vi "Export_TimeDomain_Data.vi"(0 "nCmdShow":i16(ring) items=["SW_HIDE   ", "SW_SHOWNORMAL", "SW_SHOWMINIMIZED", "SW_SHOWMAXIMIZED", "SW_SHOWNOACTIVATE", "SW_SHOW", "SW_MINIMIZE", "SW_SHOWMINNOACTIVE", "SW_SHOWNA", "SW_RESTORE"], 1 "szFileName":string="D:\\TX1.s4p", 2 "delimiterType":i16(ring) items=["Tab", "Comma"], 3 "dataFormat":i16(ring)=2 items=["StepReal", "ImpulseReal", "StepVolts", "ImpulseVolts", "StepLog", "ImpulseLog", "StepImpedance"], 4 "dataToExport":i16(ring)=3 items=["SE", "Balanced", "All ", "Customized"], 5 "stopTimeNs":dbl=3.0, 6 "ParamList":string="TDD11,TDD22", 7 "Data Points":i32=4000, 8 "Port Type":u16(ring)=1, 9 "startTimeNs":dbl, 10 "Filter?":bool, 11 "FileName":string="D:\\data.txt", 12 "Filter Risetime(ps)":dbl=50.0 min=1.0 max=1000.0 step=1.0, 13 "Compensation(ohm)":dbl=0.001 min=-20.0 max=20.0 step=0.1, 15 "Index":i32) -> (20 "Data Out":dbl[][](array[numeric]), 23 "Time Array":dbl[](array[numeric]))   [LabVIEW 2011]
uses:
  Data/Interop.PLTS.dll
  <vilib>/Utility/file.llb/Read From Spreadsheet File (DBL).vi
panel:
  out "Find?":bool=TRUE
  out "Impedance Chart":cluster{dbl[], dbl[]}[](graph)
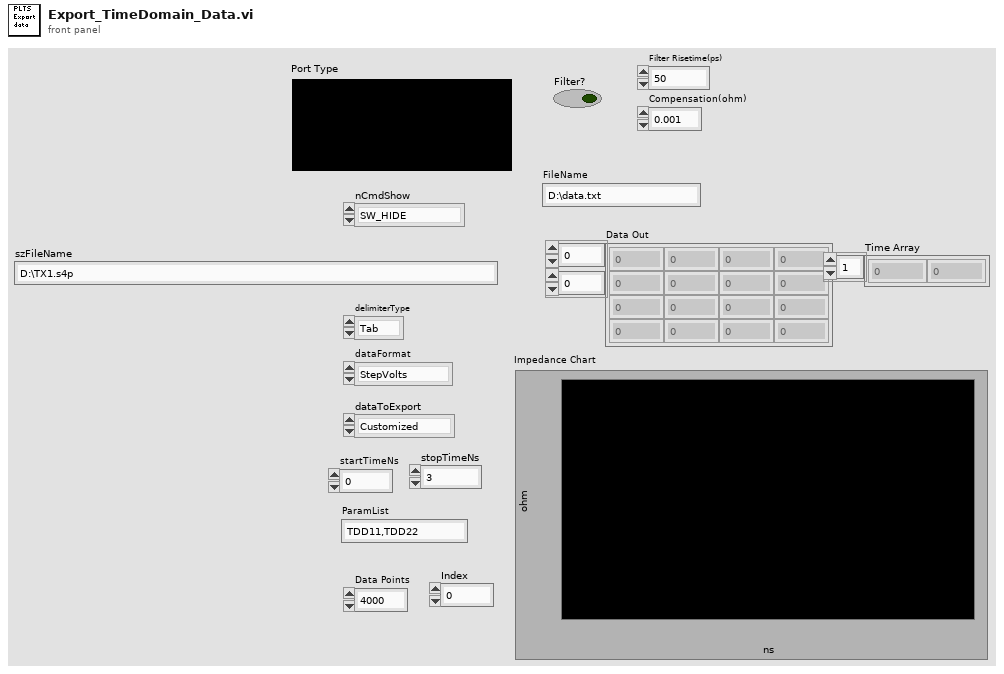
[diagram p1: front panel]
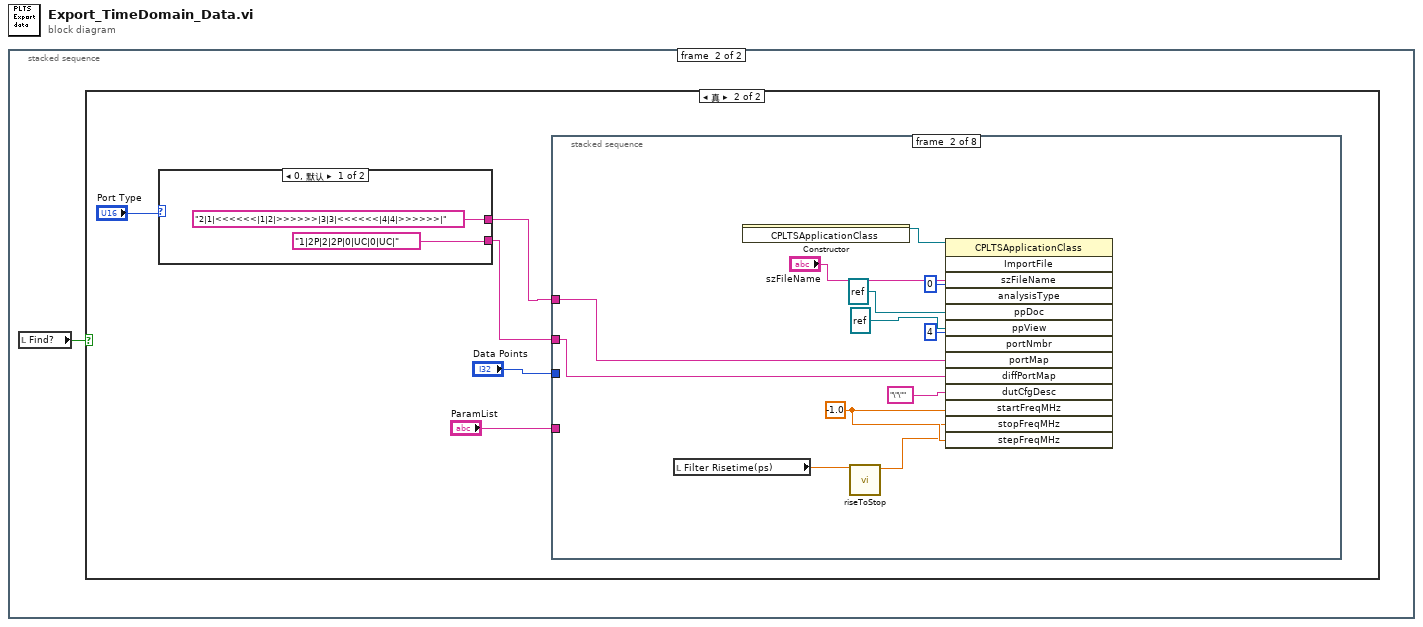
[diagram p0: block diagram]
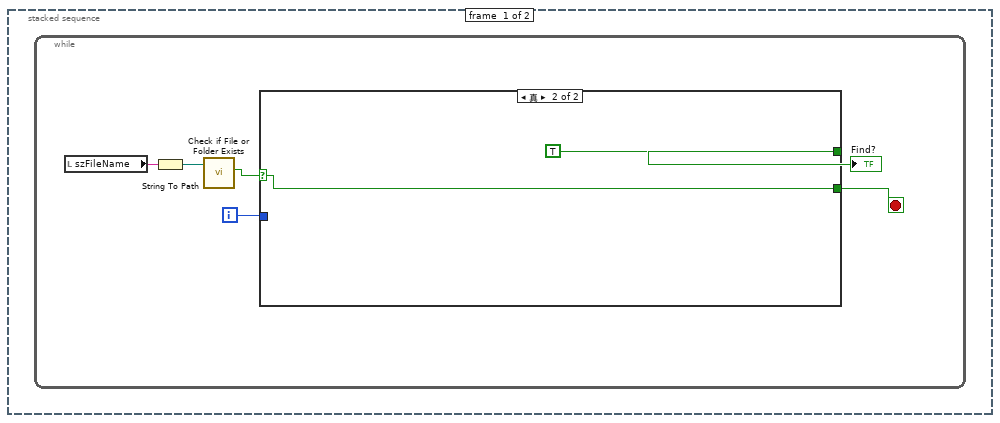
[diagram p2: hidden frame]
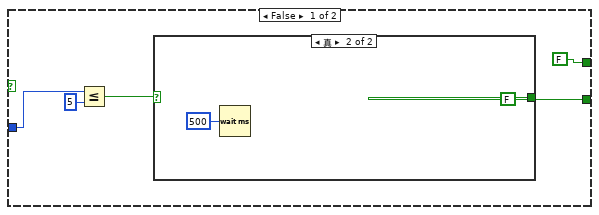
[diagram p3: hidden frame]
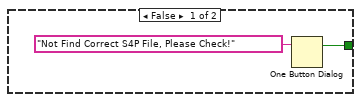
[diagram p4: hidden frame]
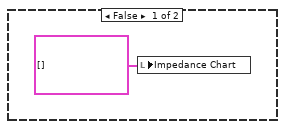
[diagram p5: hidden frame]
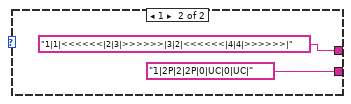
[diagram p6: hidden frame]
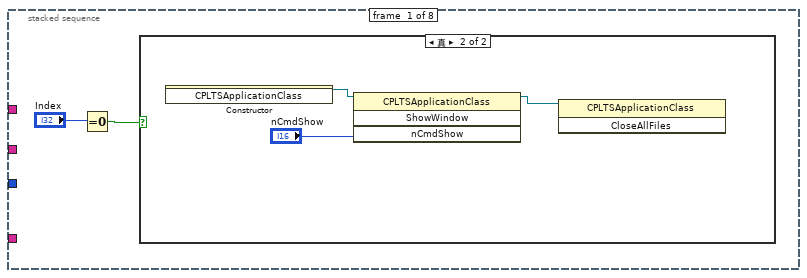
[diagram p7: hidden frame]
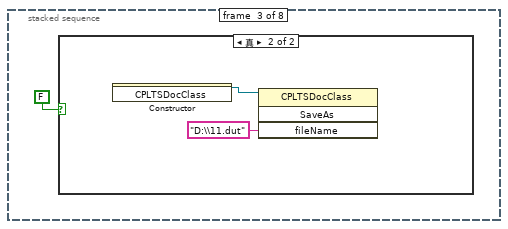
[diagram p9: hidden frame]
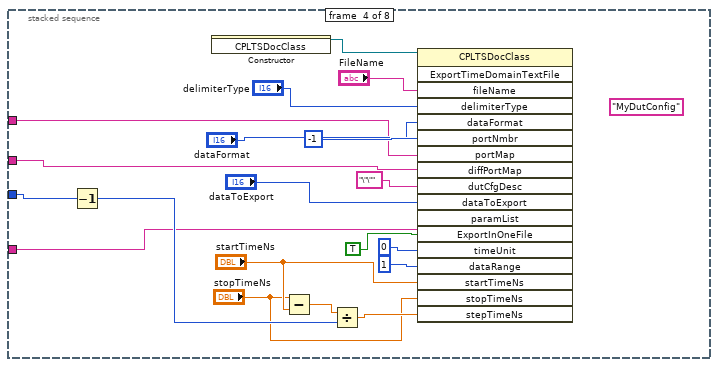
[diagram p11: hidden frame]
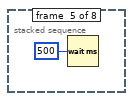
[diagram p12: hidden frame]
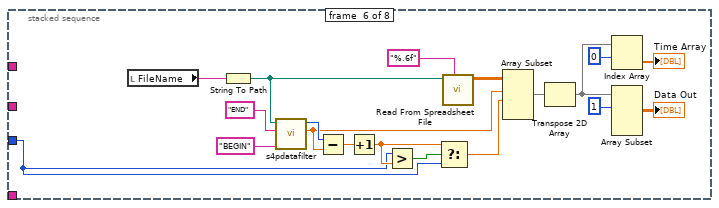
[diagram p13: hidden frame]
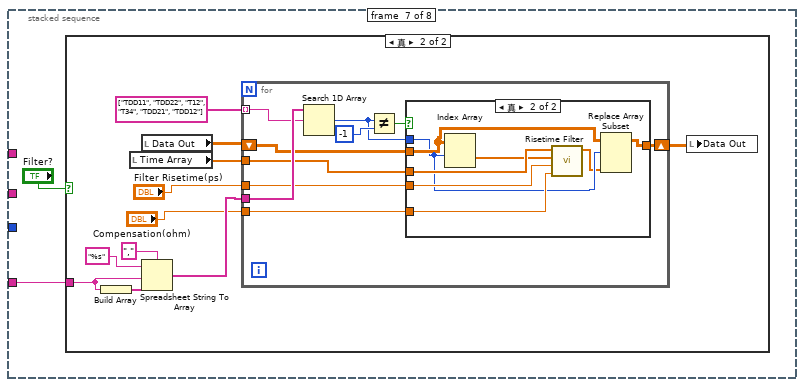
[diagram p14: hidden frame]
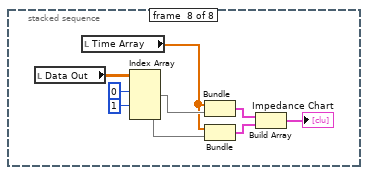
[diagram p17: hidden frame]
diagram:
  n1 = stacked-sequence {
    frame #0 {
      n2 = while {
        i -> [w2]
        stop <- w3 stop-if-true
        n3 = local read "szFileName"() -> (w6:string)
        n4 = String To Path(string=w6) -> (path=w5:path)
        n5 = call <vilib>:"Check if File or Folder Exists.vi"("path"=w5) -> ("file or folder exists?"=w4:bool)  [unwired: 8 in, 2 out]
        n6 = case shown="真" w4 {
          selector: w4 -> [_ w17]
          tunnel: [w8 w17] -> w3
          tunnel: w2 -> [w11 _]
          tunnel: [FALSE ("Find?") TRUE ("Find?")] -> w1
          frame False {
            n7 = Less Or Equal?(x=w11, y=5) -> (x <= y?=w9:bool)
            n8 = case shown="真" w9 {
              tunnel: [w13 FALSE] -> w8
              frame False {
                n9 = One Button Dialog(message="Not Find Correct S4P File, Please Check!" ("消息")) -> (true=w13:bool)  [unwired: 1 in]
              }
              frame True {
                n10 = Wait (ms)(milliseconds to wait=u32 500 ("等待时间（毫秒）")) -> ()  [unwired: 1 out]
              }
            }
          }
          frame True {
          }
        }
        "Find?" <- w1
      }
    }
    frame #1 {
      n11 = local read "Find?"() -> (w18:bool)
      n12 = case shown="真" w18 {
        frame False {
          n13 = local write "Impedance Chart"(cluster{dbl[], dbl[]}[] [] ("Impedance Chart")) -> ()
        }
        frame True {
          n14 = case shown="0, 默认" "Port Type" {
            tunnel: ["2|1|<<<<<<|1|2|>>>>>>|3|3|<<<<<<|4|4|>>>>>>|" ("portMap") "1|1|<<<<<<|2|3|>>>>>>|3|2|<<<<<<|4|4|>>>>>>|" ("portMap")] -> w21
            tunnel: ["1|2P|2|2P|0|UC|0|UC|" ("diffPortMap") "1|2P|2|2P|0|UC|0|UC|" ("diffPortMap")] -> w22
            frame 0, Default {
            }
            frame 1 {
            }
          }
          n15 = stacked-sequence {
            tunnel: "Data Points" -> [_ _ _ w57 _ w70 _ _]
            tunnel: w22 -> [_ w45 _ w54 _ _ _ _]
            tunnel: w21 -> [_ w44 _ w53 _ _ _ _]
            tunnel: "ParamList" -> [_ _ _ w49 _ _ w89 _]
            frame #0 {
              n16 = Equal To 0?(x="Index") -> (x = 0?=w29:bool)
              n17 = case shown="真" w29 {
                frame False {
                }
                frame True {
                  n18 = constructor class="CPLTSApplicationClass"() -> (reference out=w33:refnum<k24>)  [unwired: 3 in, 2 out]
                  n19 = invoke class="CPLTSApplicationClass" method="ShowWindow"(reference=w33, "nCmdShow"="nCmdShow") -> (reference out=w31:refnum<k24>)  [unwired: 2 in, 3 out]
                  n20 = invoke class="CPLTSApplicationClass" method="CloseAllFiles"(reference=w31) -> ()  [unwired: 2 in, 3 out]
                }
              }
            }
            frame #1 {
              w37 = -1.0 ("startFreqMHz")
              n21 = local read "Filter Risetime(ps)"() -> (w34:dbl)
              n22 = constructor class="CPLTSApplicationClass"() -> (reference out=w43:refnum<k24>)  [unwired: 3 in, 2 out]
              n23 = call "riseToStop.vi"("riseTime"=w34) -> ("stopFre"=w35:dbl)  [unwired: 10 in]
              n24 = invoke class="CPLTSApplicationClass" method="ImportFile"(reference=w43, "szFileName"="szFileName", "analysisType"=i16 0, "ppDoc"=refnum<k24> refnum, "ppView"=refnum<k24> refnum, "portNmbr"=i16 4, "portMap"=w44, "diffPortMap"=w45, "dutCfgDesc"="\"\"" ("portMap"), "startFreqMHz"=w37, "stopFreqMHz"=w35, "stepFreqMHz"=w37) -> ()  [unwired: 2 in, 14 out]
            }
            frame #2 {
              n25 = case shown="真" FALSE {
                frame False {
                }
                frame True {
                  n26 = constructor class="CPLTSDocClass"() -> (reference out=w48:refnum<k24>)  [unwired: 3 in, 2 out]
                  n27 = invoke class="CPLTSDocClass" method="SaveAs"(reference=w48, "fileName"="D:\\11.dut") -> ()  [unwired: 2 in, 4 out]
                }
              }
            }
            frame #3 {
              (unwired) "MyDutConfig" ("dutCfgDesc")
              n28 = Decrement(x=w57) -> (x-1=w56:i32)
              n29 = constructor class="CPLTSDocClass"() -> (reference out=w67:refnum<k24>)  [unwired: 3 in, 2 out]
              n30 = Subtract(x="stopTimeNs", y="startTimeNs") -> (x-y=w51:dbl)
              n31 = Divide(x=w51, y=w56) -> (x/y=w59:dbl)
              n32 = invoke class="CPLTSDocClass" method="ExportTimeDomainTextFile"(reference=w67, "fileName"="FileName", "delimiterType"="delimiterType", "dataFormat"="dataFormat", "portNmbr"=i16 -1, "portMap"=w53, "diffPortMap"=w54, "dutCfgDesc"="\"\"" ("portMap"), "dataToExport"="dataToExport", "paramList"=w49, "ExportInOneFile"=TRUE, "timeUnit"=i16 0, "dataRange"=i16 1, "startTimeNs"="startTimeNs", "stopTimeNs"="stopTimeNs", "stepTimeNs"=w59) -> ()  [unwired: 2 in, 18 out]
            }
            frame #4 {
              n33 = Wait (ms)(milliseconds to wait=u32 500 ("等待时间（毫秒）")) -> ()  [unwired: 1 out]
            }
            frame #5 {
              n34 = local read "FileName"() -> (w87:string)
              n35 = String To Path(string=w87) -> (path=w78:path)
              n36 = call "s4pdatafilter.vi"("Begin"="BEGIN", "End"="END", "file path (dialog if empty)"=w78) -> ("begin"=w74:dbl, "end"=w75:i32)  [unwired: 7 in]
              n37 = Subtract(x=w75, y=w74) -> (x-y=w73:dbl)
              n38 = Increment(x=w73) -> (x+1=w71:dbl)
              n39 = Greater?(x=w70, y=w71) -> (0:w72:bool)
              n40 = Select(t=w71, s=w72, f=w70) -> (s? t:f=w69:dbl)
              n41 = call-poly <vilib>:"Read From Spreadsheet File.vi"("format (%.3f)"="%.6f", "file path (dialog if empty)"=w78) -> ("all rows"=w79:dbl[][])  [unwired: 5 in, 4 out]
              n42 = Array Subset(array=w79, index (row)=w74, length (row)=w69) -> (w80:dbl[][])  [unwired: 2 in]
              n43 = Transpose 2D Array(2D array=w80) -> (transposed array=w83:dbl[][])
              n44 = Index Array(array=w83, index (row)=0 ("索引 (行)")) -> (element=→"Time Array":dbl[])  [unwired: 1 in]
              n45 = Array Subset(array=w83, index (row)=1 ("索引")) -> (→"Data Out":dbl[][])  [unwired: 3 in]
            }
            frame #6 {
              n46 = case shown="真" "Filter?" {
                tunnel: w89 -> [_ w98]
                frame False {
                }
                frame True {
                  n47 = Build Array(w98) -> (w97:string[])
                  n48 = local read "Time Array"() -> (w93:dbl[])
                  n49 = local read "Data Out"() -> (w95:dbl[][])
                  n50 = Spreadsheet String To Array(delimiter (Tab)="," ("分隔符(Tab)"), format string="%s" ("格式字符串"), spreadsheet string=w98, array type (2D Dbl)=w97) -> (array=w94:string[])
                  n51 = for {
                    tunnel: string[] ["TDD11", "TDD22", "T12", "T34", "TDD21", "TDD12"] ("Selected Time item") -> [w109] mode=indexing
                    shift-right: [w102] -> w90
                    shift-left: w95 -> [w106]
                    tunnel: w94 -> [w110]
                    tunnel: w93 -> [w108]
                    tunnel: "Filter Risetime(ps)" -> [w104]
                    tunnel: "Compensation(ohm)" -> [w103]
                    n52 = Search 1D Array(1D array=w110, element=w109) -> (index of element=w101:i32)  [unwired: 1 in]
                    n53 = Not Equal?(x=w101, y=-1) -> (x != y?=w107:bool)
                    n54 = case shown="真" w107 {
                      tunnel: w108 -> [_ w119]
                      tunnel: w106 -> [w111 w114]
                      tunnel: w101 -> [_ w113]
                      tunnel: w104 -> [_ w117]
                      tunnel: w103 -> [_ w116]
                      tunnel: [w111 w115] -> w102
                      frame False {
                      }
                      frame True {
                        n55 = Index Array(array=w114, index (row)=w113) -> (element=w118:dbl[])  [unwired: 1 in]
                        n56 = call "Risetime Filter.vi"("Compensation(ohm)"=w116, "Filter Risetime(ps)"=w117, "Data in"=w118, "Time Axis"=w119) -> ("Data Out"=w112:dbl[])  [unwired: 7 in]
                        n57 = Replace Array Subset(array=w114, new element=w112, index (row)=w113) -> (w115:dbl[][])  [unwired: 1 in]
                      }
                    }
                  }
                  n58 = local write "Data Out"(w90) -> ()
                }
              }
            }
            frame #7 {
              n59 = local read "Data Out"() -> (w124:dbl[][])
              n60 = local read "Time Array"() -> (w123:dbl[])
              n61 = Index Array(array=w124, index (row) #1=0 ("索引 (行)"), index (row) #2=1 ("索引 (列)")) -> (element #1=w127:dbl[], element #2=w128:dbl[])  [unwired: 2 in]
              n62 = Bundle("Time Array"=w123, "Data Out"=w127) -> (w122:cluster{"Time Array":dbl[], "Data Out":dbl[]})  [unwired: 1 in]
              n63 = Bundle("Time Array"=w123, "Data Out"=w128) -> (w120:cluster{"Time Array":dbl[], "Data Out":dbl[]})  [unwired: 1 in]
              n64 = Build Array(w122, w120) -> (→"Impedance Chart":cluster{"Time Array":dbl[], "Data Out":dbl[]}[])
            }
          }
        }
      }
    }
  }
